vi "LSCI332 GetSetPoint.vi"(0 "VISA Rsrc":refnum<visa-resource-name>="GPIB0::12::INSTR", 5 "Boucle(1)":u32(ring) caption="Boucle" items=["Boucle 1", "Boucle 2"], 11 "error in (no error)":errorcluster) -> (4 "SetPoint":dbl, 15 "error out":errorcluster)   [LabVIEW 2019]
doc: "Ce VI lit les paramètres limites de contrôle et ceux de stabilisation du contrôleur."
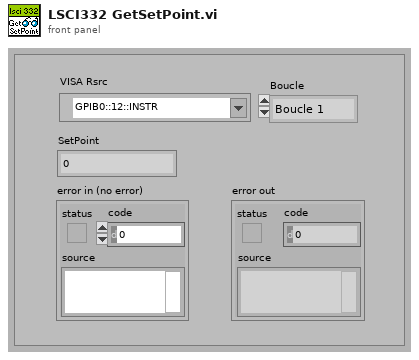
[diagram p1: front panel]
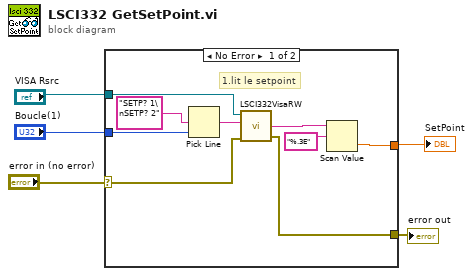
[diagram p0: block diagram]
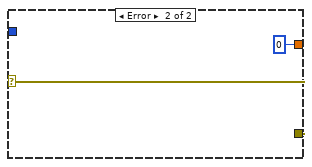
[diagram p2: hidden frame]
diagram:
  n1 = case shown="No Error" "error in (no error)" {
    selector: "error in (no error)" -> [w13 w16]
    tunnel: "VISA Rsrc" -> [w14 _]
    tunnel: "Boucle(1)" -> [w11 _]
    tunnel: [w9 w16] -> w3
    tunnel: [w7 u32 0] -> w1
    frame No Error {
      # "1.lit le setpoint"
      n2 = Pick Line(multi-line string="SETP? 1\nSETP? 2", line index=w11) -> (output string=w10:string)  [unwired: 1 in]
      n3 = call <userlib>:"LSCI332VisaRW.vi"("error in (no error)"=w13, "ChaineCom"=w10, "VISA Rsrc"=w14) -> ("error out"=w9:errorcluster, "ChaineRep"=w8:string)  [unwired: 4 in, 2 out]
      n4 = Scan Value(string=w8, format string="%.3E") -> (value=w7:dbl)  [unwired: 1 in, 1 out]
    }
    frame Error {
    }
  }
  "error out" <- w3
  "SetPoint" <- w1
